vi "setCommandEvents.vi"(8 "error in (no error)":errorcluster, 10 "Tools.lvlib:Interpreters.lvlib:CommandEvents.lvclass":refnum<class "CommandEvents.lvclass">, 11 "ConsoleViewer.lvclass in":refnum<class "ConsoleViewer.lvclass">) -> (0 "error out":errorcluster, 3 "ConsoleViewer.lvclass out":refnum<class "ConsoleViewer.lvclass">)   [LabVIEW 2009, in "Views.lvlib" / "ConsoleViewer.lvclass"]
uses:
  ConsoleViewer.lvclass
  Tools/CommandProcessor/CommandEvents/CommandEvents.lvclass
  ConsoleViewer.lvclass/ConsoleViewer.ctl
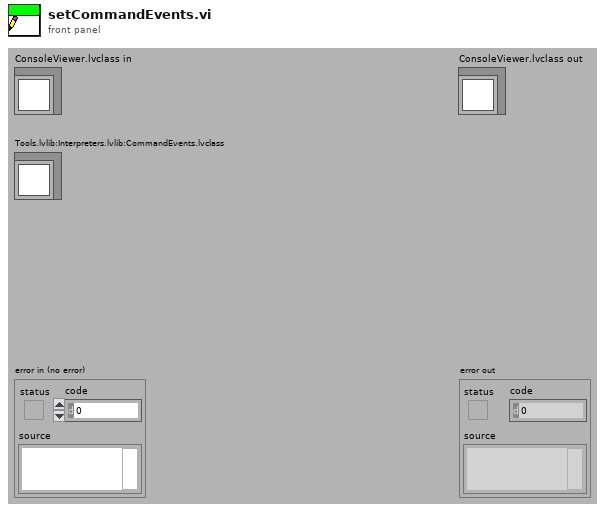
[diagram p1: front panel]
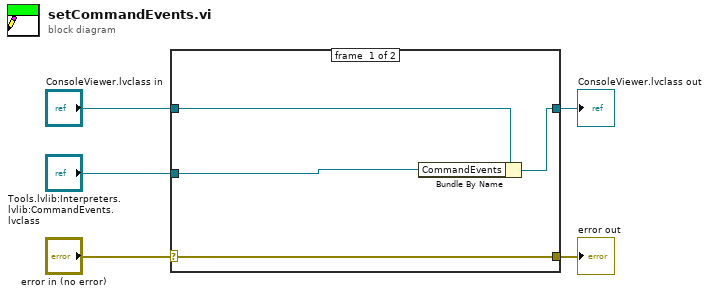
[diagram p0: block diagram]
diagram:
  n1 = case shown="No Error" "error in (no error)" {
    selector: "error in (no error)" -> [w9 w10]
    tunnel: [w9 w10] -> w4
    tunnel: [w7 w11] -> w2
    tunnel: "ConsoleViewer.lvclass in" -> [w8 w11]
    tunnel: "Tools.lvlib:Interpreters.lvlib:CommandEvents.lvclass" -> [w6 _]
    frame #0 {
      n2 = Bundle By Name(cluster=w8, "CommandEvents"=w6) -> (w7:refnum<class "ConsoleViewer.lvclass">)
    }
    frame #1 {
    }
  }
  "error out" <- w4
  "ConsoleViewer.lvclass out" <- w2
